vi "Write Header and Times.vi"(0 "Cells Hz IN":refnum<k7>, 5 "Cells Ave IN":refnum<k7>, 7 "Header Array":string[](array[string]), 9 "Time Array":string[](array[string]), 11 "Ave.ingLength":i32) -> (4 "Cells Hz OUT":refnum<k7>, 6 "Cells Ave OUT":refnum<k7>)   [LabVIEW 2019]
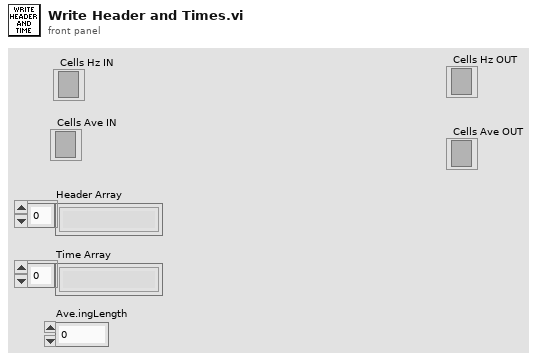
[diagram p1: front panel]
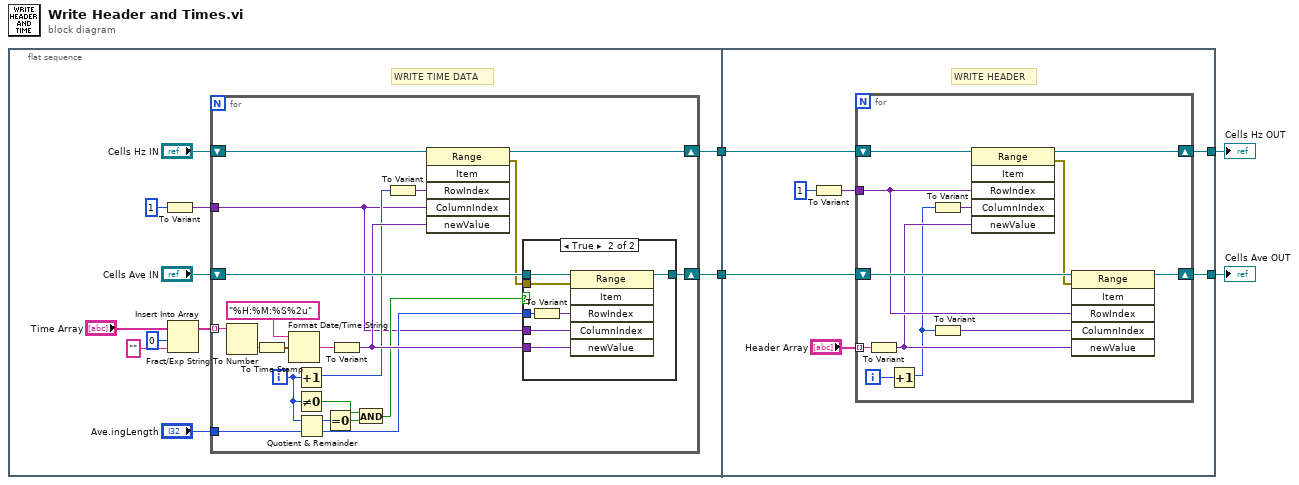
[diagram p0: block diagram]
diagram:
  n1 = flat-sequence {
    tunnel: [w6] -> w4
    tunnel: [w5] -> w3
    tunnel: w4 -> [w48]
    tunnel: w3 -> [w47]
    tunnel: [w46] -> w2
    tunnel: [w45] -> w1
    frame #0 {
      # "WRITE TIME DATA"
      n2 = To Variant(anything=1) -> (Variant=w8:variant)
      n3 = Insert Into Array(array="Time Array", index=0, new element="" ("String")) -> (w14:string[])
      n4 = for {
        tunnel: w14 -> [w20] mode=indexing
        tunnel: w8 -> [w24]
        tunnel: "Ave.ingLength" -> [w32]
        shift-right: [w18] -> w6
        shift-left: "Cells Hz IN" -> [w35]
        shift-right: [w17] -> w5
        shift-left: "Cells Ave IN" -> [w36]
        i -> [w31]
        n5 = Fract/Exp String To Number(string=w20) -> (number=w21:dbl)  [unwired: 3 in, 1 out]
        n6 = To Time Stamp(1:w21) -> (0:w23:timestamp)
        n7 = Format Date/Time String(time format string (%c)="%H:%M:%S%2u", seconds (now)=w23) -> (date/time string=w19:string)  [unwired: 1 in]
        n8 = Increment(x=w31) -> (x+1=w33:i32)
        n9 = Not Equal To 0?(x=w31) -> (x != 0?=w28:bool)
        n10 = Quotient & Remainder(x=w31, y=w32) -> (x-y*floor(x/y)=w30:i32, floor(x/y)=w26:i32)
        n11 = Equal To 0?(x=w30) -> (x = 0?=w29:bool)
        n12 = To Variant(anything=w19) -> (Variant=w34:variant)
        n13 = And(x=w28, y=w29) -> (x .and. y?=w27:bool)
        n14 = To Variant(anything=w33) -> (Variant=w25:variant)
        n15 = invoke class="Range" method="Item"(reference=w35, "RowIndex"=w25, "ColumnIndex"=w24, "newValue"=w34) -> (reference out=w18:refnum<k7>, error out=w16:errorcluster)  [unwired: 2 in, 4 out]
        n16 = case shown="True" w27 {
          tunnel: w36 -> [w37 w44]
          tunnel: w34 -> [_ w43]
          tunnel: w26 -> [_ w42]
          tunnel: w24 -> [_ w40]
          tunnel: [w37 w39] -> w17
          tunnel: w16 -> [_ w38]
          frame False {
          }
          frame True {
            n17 = To Variant(anything=w42) -> (Variant=w41:variant)
            n18 = invoke class="Range" method="Item"(reference=w44, error in=w38, "RowIndex"=w41, "ColumnIndex"=w40, "newValue"=w43) -> (reference out=w39:refnum<k7>)  [unwired: 1 in, 5 out]
          }
        }
      }
    }
    frame #1 {
      # "WRITE HEADER"
      n19 = To Variant(anything=1) -> (Variant=w49:variant)
      n20 = for {
        tunnel: "Header Array" -> [w59] mode=indexing
        tunnel: w49 -> [w60]
        shift-right: [w53] -> w46
        shift-left: w48 -> [w61]
        shift-right: [w54] -> w45
        shift-left: w47 -> [w62]
        i -> [w57]
        n21 = To Variant(anything=w59) -> (Variant=w58:variant)
        n22 = Increment(x=w57) -> (x+1=w55:i32)
        n23 = To Variant(anything=w55) -> (Variant=w63:variant)
        n24 = To Variant(anything=w55) -> (Variant=w56:variant)
        n25 = invoke class="Range" method="Item"(reference=w61, "RowIndex"=w60, "ColumnIndex"=w63, "newValue"=w58) -> (reference out=w53:refnum<k7>, error out=w52:errorcluster)  [unwired: 2 in, 4 out]
        n26 = invoke class="Range" method="Item"(reference=w62, error in=w52, "RowIndex"=w60, "ColumnIndex"=w56, "newValue"=w58) -> (reference out=w54:refnum<k7>)  [unwired: 1 in, 5 out]
      }
    }
  }
  "Cells Hz OUT" <- w2
  "Cells Ave OUT" <- w1
